vi "Remove Group.vi"(8 "error in (no error)":errorcluster, 11 "BluelinesRedlines in":refnum<class "BluelinesRedlines.lvclass">) -> (0 "error out":errorcluster, 3 "BluelinesRedlines out":refnum<class "BluelinesRedlines.lvclass">)   [LabVIEW 2020, in "VolatusGUIElements.lvlib" / "BluelinesRedlines.lvclass"]
uses:
  BluelinesRedlines.lvclass
  BluelinesRedlines.lvclass/BluelinesRedlines.ctl
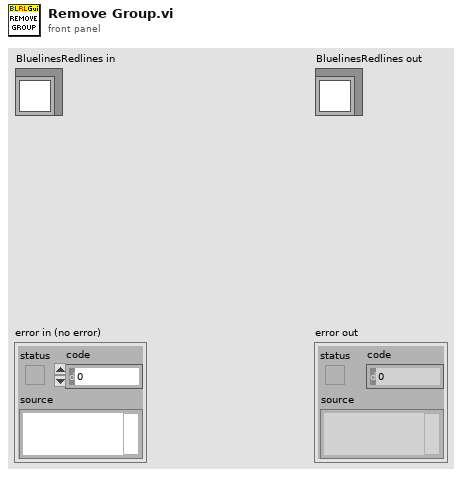
[diagram p1: front panel]
types:
  T1 = map{string, refnum<class "BluelinesRedlines Source.lvclass">}
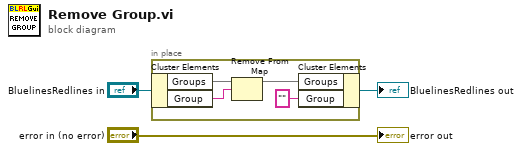
[diagram p0: block diagram]
diagram:
  n1 = in-place {
    n2 = in-place-cluster #1("BluelinesRedlines in") -> ("Groups"=w7:T1, "Group"=w6:string)
    n3 = Remove From Map(10:w6, 11:w7) -> (3:w5:T1)  [unwired: 2 out]
    n4 = in-place-cluster #1("Groups"=w5, "Group"="") -> (→"BluelinesRedlines out":refnum<class "BluelinesRedlines.lvclass">)
  }
  "error out" <- "error in (no error)"
